vi "Check if Initialized.vi"(8 "error in (no error)":errorcluster, 11 "Process in":refnum<class "Process.lvclass">) -> (0 "error out":errorcluster, 2 "Initialized?":bool, 3 "Process out":refnum<class "Process.lvclass">)   [LabVIEW 2020, in "Process.lvclass"]
uses:
  Process.lvclass
  Process.lvclass/Process.ctl
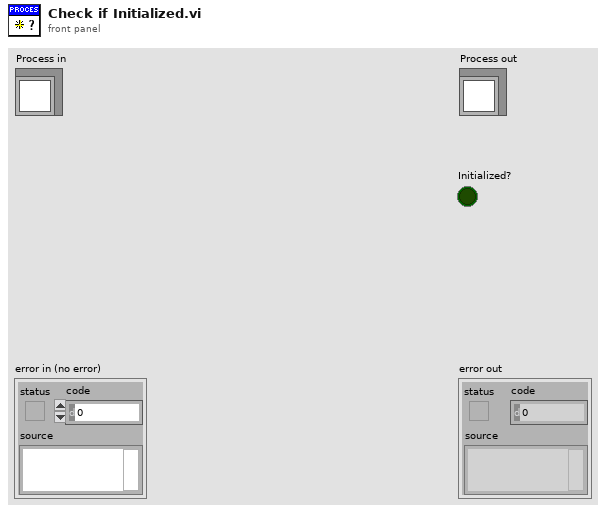
[diagram p1: front panel]
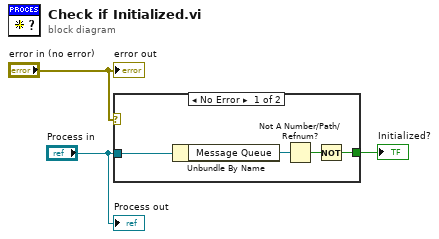
[diagram p0: block diagram]
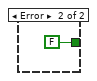
[diagram p2: hidden frame]
diagram:
  n1 = case shown="No Error" "error in (no error)" {
    tunnel: "Process in" -> [w7 _]
    tunnel: [w4 FALSE] -> w2
    frame No Error {
      n2 = Unbundle By Name(w7) -> ("Message Queue"=w6:refnum<queue>)
      n3 = Not A Number/Path/Refnum?(number/path/refnum=w6) -> (NaN/Path/Refnum?=w5:bool)
      n4 = Not(x=w5) -> (.not. x?=w4:bool)
    }
    frame Error {
    }
  }
  "Initialized?" <- w2
  "error out" <- "error in (no error)"
  "Process out" <- "Process in"
